vi "Send Command.vi"(8 "error in (no error)":errorcluster, 10 "Parameter":variant, 11 "Command":T1) -> (0 "error out":errorcluster)   [LabVIEW 2016]
uses:
  HostRTCommunication/Commands.ctl
  HostRTCommunication/Command and Parameters.ctl
  Application Control/Application Globals.vi
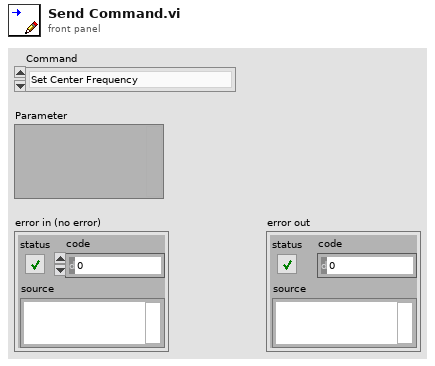
[diagram p1: front panel]
types:
  T1 = typedef "Commands.ctl" = enum16{"Set Center Frequency", "Set AGC State", "Set Number Of Averages", "Set Tuner Gain Mode", "Set Frequency Correction", "Set Sample Rate", "Set Manual Gain Value"}
  T2 = typedef "Command and Parameters.ctl" = cluster{"Command":T1, "Command Parameters":variant[]}
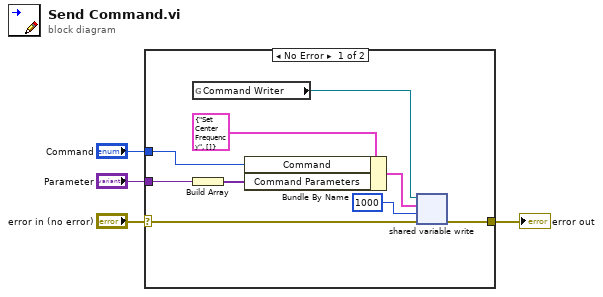
[diagram p0: block diagram]
diagram:
  n1 = case shown="No Error" "error in (no error)" {
    selector: "error in (no error)" -> [w6 w14]
    tunnel: [w13 w14] -> w4
    tunnel: "Parameter" -> [w9 _]
    tunnel: "Command" -> [w7 _]
    frame No Error {
      n2 = global read "Application Globals.vi" "Command Writer"() -> (w12:refnum<k21>)
      n3 = Build Array(w9) -> (w8:variant[])
      n4 = Bundle By Name(cluster=T2 {"Command"=enum."Set Center Frequency", "Command Parameters"=[]} ("Cluster"), "Command"=w7, "Command Parameters"=w8) -> (w10:T2)
      n5 = shared-variable-write(w12, w6, w10, 1000 ("timeout ms (-1)")) -> (w13:errorcluster)  [unwired: 2 out]
    }
    frame Error {
    }
  }
  "error out" <- w4
